vi "Remove Outliers.vi"   [LabVIEW 2016, in "xy_utilities.lvlib"]
doc: "Remove outliers from the y array of <b>XY-data</b> between <b>Y Upper</b> and <b>Y Lower</b> limits.\n\nWire data to the data input to determine the polymorphic instance to use or manually select the instance."
uses:
  xy_utilities.lvlib
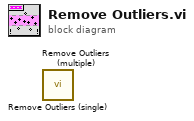
[diagram p0: block diagram]
diagram:
  n1 = call "Remove Outliers (single).vi"() -> ()  [unwired: 10 in, 2 out]
  n2 = call "Remove Outliers (multiple).vi"() -> ()  [unwired: 10 in, 2 out]
